vi "Update Message log.vi"(8 "error in (no error)":errorcluster, 10 "New Message":string, 11 "Chat Window UI in":refnum<class "Chat Window Controller UI.lvclass">) -> (0 "error out":errorcluster, 3 "Chat Window UI out":refnum<class "Chat Window Controller UI.lvclass">)   [LabVIEW 2020, in "Chat Window UI.lvlib" / "Chat Window Controller UI.lvclass"]
uses:
  Chat Window Controller UI.lvclass
  Chat Window Controller UI.lvclass/Chat Window Controller UI.ctl
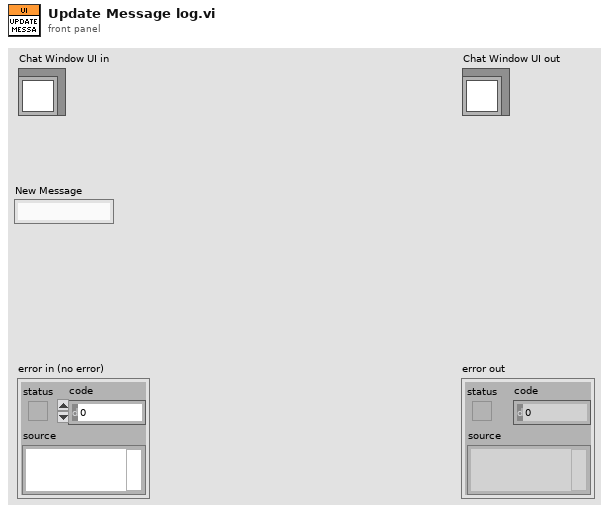
[diagram p1: front panel]
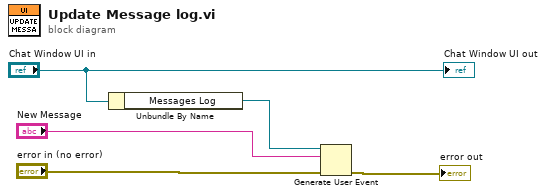
[diagram p0: block diagram]
diagram:
  n1 = Unbundle By Name("Chat Window UI in") -> ("Messages Log"=w4:refnum<user-event>)
  n2 = Generate User Event(user event=w4, event data cluster="New Message", error in="error in (no error)") -> (error out=→"error out":errorcluster)  [unwired: 1 in, 1 out]
  "Chat Window UI out" <- "Chat Window UI in"
